vi "Top Level FPGA.vi"() -> ()   [LabVIEW 2012]
uses:
  <vilib>/Platform/TimedLoop/XDataNode/XDataNode.xnode
  <vilib>/Platform/TimedLoop/XDataNode/nitl_modes.ctl
  <vilib>/Platform/TimedLoop/XDataNode/XDNodeRunTimeDep.lvlib
  <vilib>/Platform/TimedLoop/XDataNode/wakeup.ctl
  <vilib>/Platform/TimedLoop/XDataNode/timing_clust.ctl
  <vilib>/rvi/DataTransferAndStorage/Container/Common/niFpgaContainerMetaDataKey.ctl
  <vilib>/rvi/FIFO/Fifo_Types/niFpgaFifoControlLogicControl.ctl
  <vilib>/rvi/Memory/Memory_Types/niFpgaMemoryInterfaceConfiguration.ctl
  <vilib>/rvi/DataTransferAndStorage/Container/Common/niFpgaContainerInitializationParameters.ctl
  <vilib>/rvi/DataTransferAndStorage/Container/Common/niFpgaTransferTypeControl.ctl
  <vilib>/rvi/DataTransferAndStorage/Container/Common/niFpgaContainerArbitrationOptionsControl.ctl
  <vilib>/rvi/DataTransferAndStorage/Container/Common/niFpgaContainerImplementationControl.ctl
  <vilib>/rvi/DataTransferAndStorage/Container/Common/niFpgaDataTypeControl.ctl
  <vilib>/rvi/DataTransferAndStorage/Container/Common/niFpgaContainerState.ctl
  <vilib>/rvi/DataTransferAndStorage/Container/Common/niFpgaContainerSetEmuInfo.vi
  <vilib>/rvi/eio/common/nirviEmuReportErrorAndStop.vi
  <vilib>/rvi/DataTransferAndStorage/Container/Common/niFpgaContainerGetUniqueNameForEmu.vi
  <vilib>/rvi/LocalResourceManager/LocalResourceManager.xnode
  <vilib>/rvi/DataTransferAndStorage/Container/XNode/niFpgaContainer.xnode
  <vilib>/rvi/Memory/Memory_Emulation/nirvimemoryEmulation.vi
  <vilib>/rvi/FIFO/Fifo_Resource/nirvififoEmulationRead.vi
  <vilib>/rvi/FIFO/Fifo_Resource/nirvififoEmulationWrite.vi
  <vilib>/rvi/DataTransferAndStorage/Register/Emulation/niFpgaRegisterEmulation.vi
  <vilib>/eio/EIONode/EIONode.xnode
  <vilib>/rvi/eio/common/nirviEmuTemplateMethod_errors.vi
panel:
  in  "# of pretrigger":u32
  out "IO Module\\Pll Unlocked":bool
  out "IO Module\\ADC Error B":bool
  out "IO Module\\ADC Error A":bool
  out "Init Done":bool
  in  "Simulate":bool
  in  "Trigger 5":i16=12500
  in  "Trigger 6":i16=12500
  in  "Trigger 7":i16=12500
  in  "Trigger 8":i16=12500
  in  "Trigger 3":i16=12500
  in  "Trigger 4":i16=12500
  in  "Trigger 2":i16=12500
  in  "Record Size":u32=300
  in  "Trigger 1":i16=12500
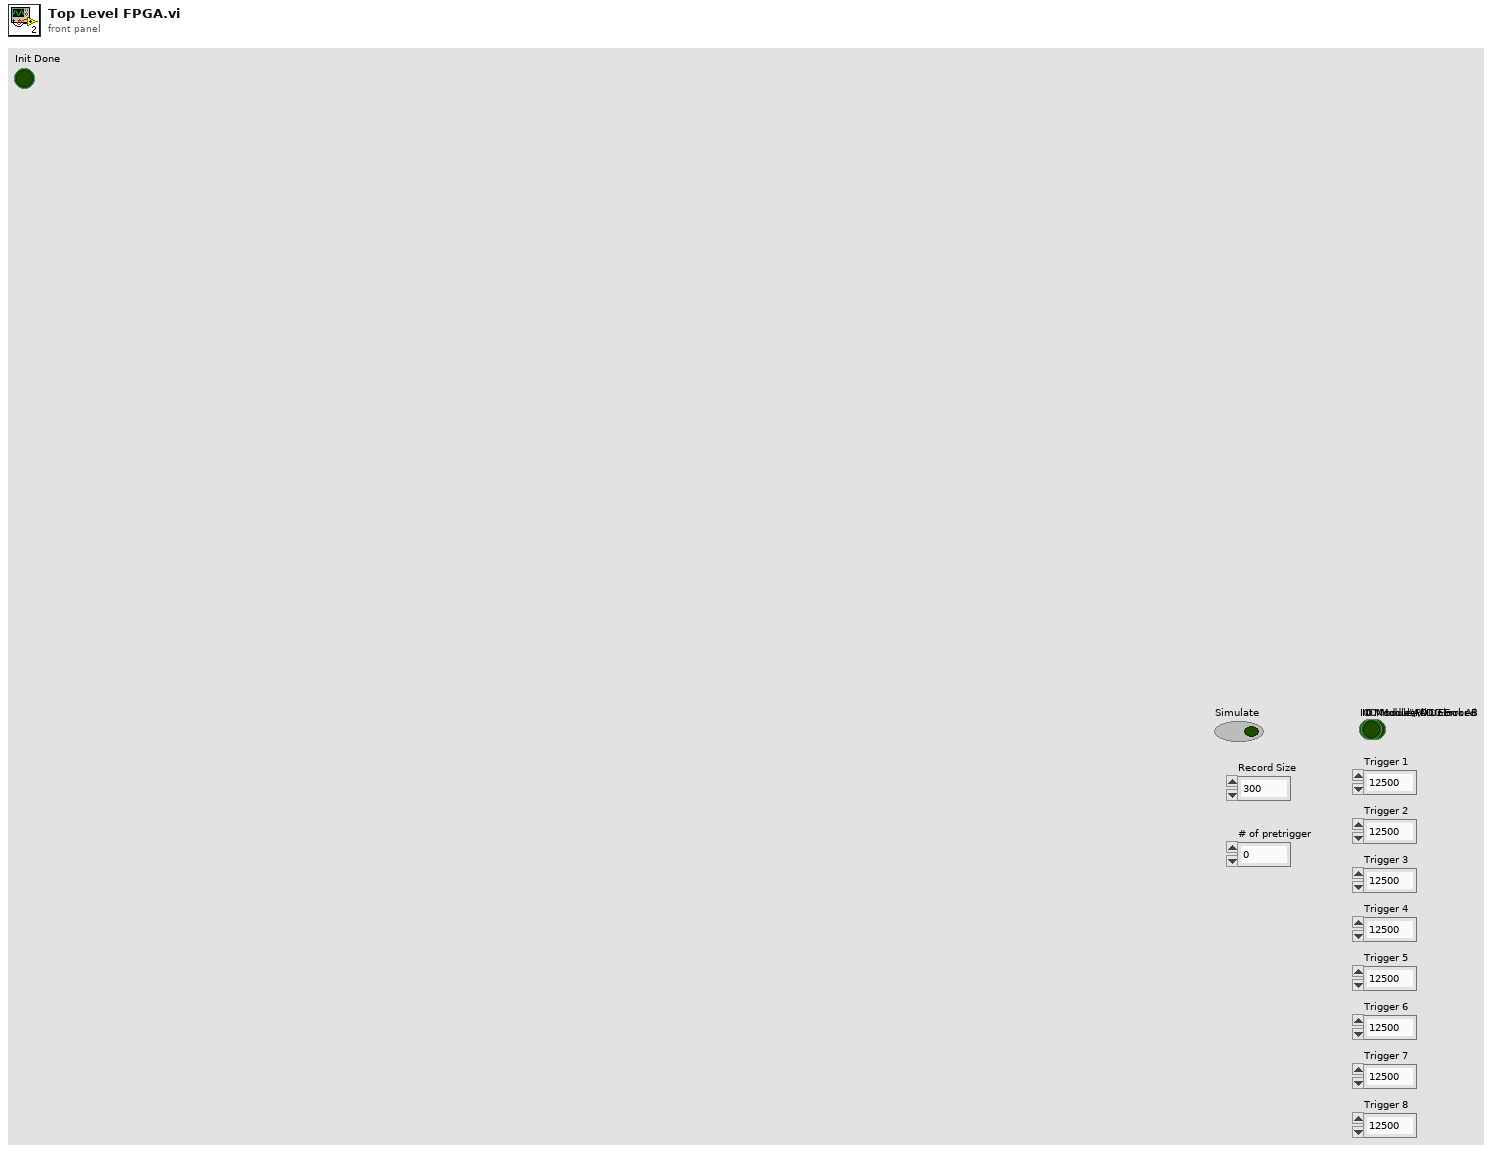
[diagram p1: front panel]
types:
  T1 = typedef "XDNodeRunTimeDep.lvlib/timing_clust.ctl" = cluster{"Expected End [f-1]":u64, "Actual End [f-1]":u64, "Finished Late? [f-1]":bool, "Expected End [i-1]":u64, "Actual End [i-1]":u64, "Finished Late? [i-1]":bool, "Expected Start [i]":u64, "Actual Start [i]":u64, "Expected Start [f]":u64, "Actual Start [f]":u64, "Source Name":string, "Structure Name":string, "Period":i64, "Deadline":i64, "Offset":i64, "Start":i64, "Priority":i32, "Timeout":i32, "Mode":T2, "Wakeup Reason":T3, "Error":errorcluster, "Source Type":string, "Secondary Source Type":string, "Global End Time":u64, "Global Start Time":u64, "Frame Duration":u64, "Iteration Duration":u64, "Assigned CPU":i32, "I/O Scan Engine Mode":u32}
  T2 = typedef "XDNodeRunTimeDep.lvlib/nitl_modes.ctl" = enum32{"No Change", "Process missed periods, maintain original phase", "Discard missed periods, maintain original phase", "Process missed periods, ignore original phase", "Discard missed periods, ignore original phase"}
  T3 = typedef "XDNodeRunTimeDep.lvlib/wakeup.ctl" = enum32{"Normal", "Aborted", "Asynchronous wakeup", "Timing source error", "Timed loop error", "Timeout"}
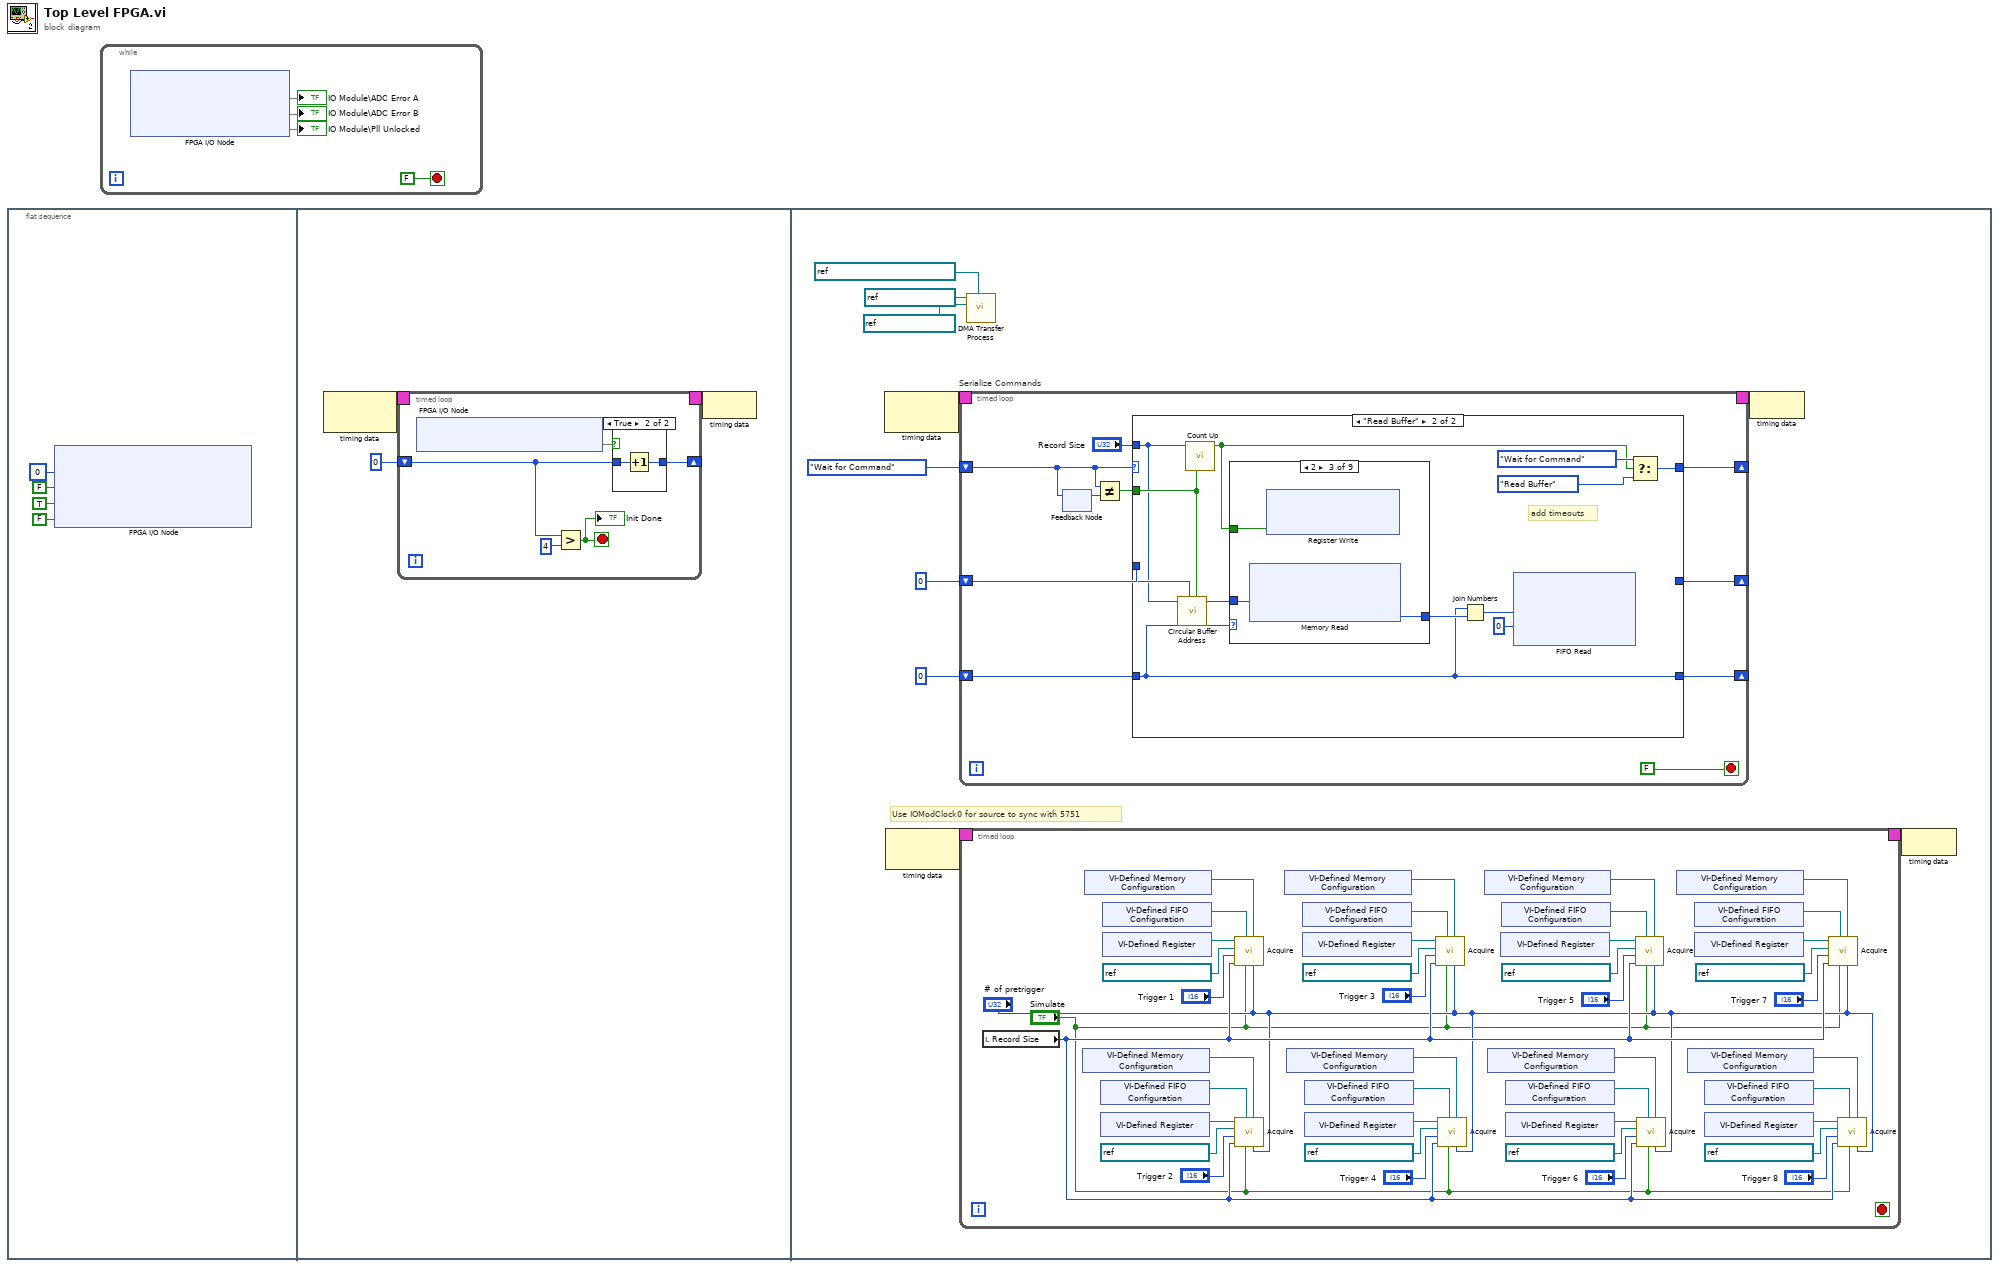
[diagram p0: block diagram]
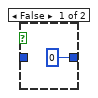
[diagram p2: hidden frame]
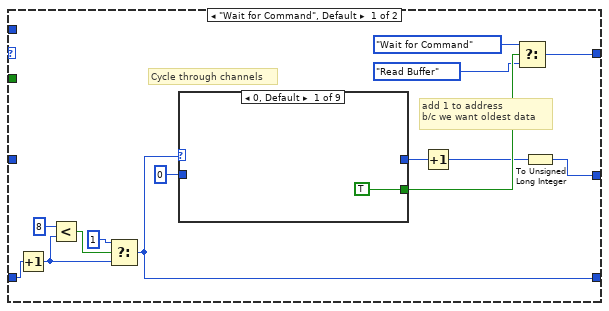
[diagram p3: hidden frame]
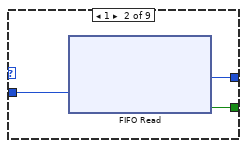
[diagram p4: hidden frame]
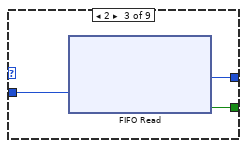
[diagram p5: hidden frame]
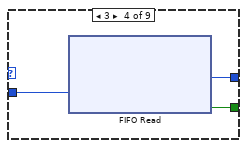
[diagram p6: hidden frame]
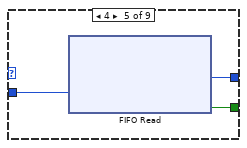
[diagram p7: hidden frame]
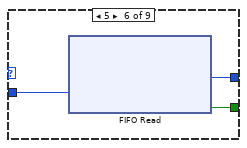
[diagram p8: hidden frame]
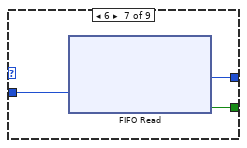
[diagram p9: hidden frame]
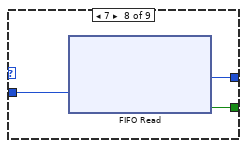
[diagram p10: hidden frame]
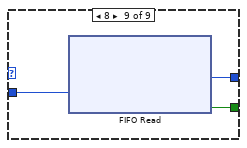
[diagram p11: hidden frame]
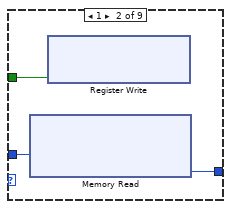
[diagram p13: hidden frame]
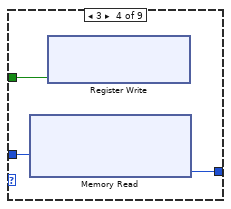
[diagram p14: hidden frame]
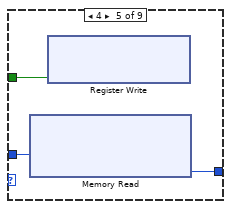
[diagram p15: hidden frame]
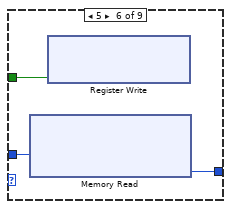
[diagram p16: hidden frame]
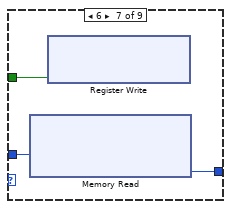
[diagram p17: hidden frame]
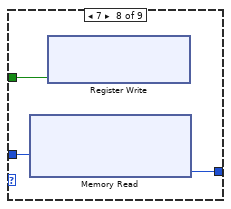
[diagram p18: hidden frame]
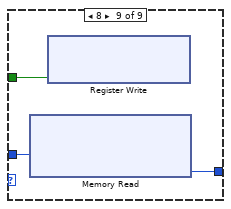
[diagram p19: hidden frame]
diagram:
  n1 = flat-sequence {
    frame #0 {
      n2 = xnode "FPGA I/O Node"("IO Module\\Sample Clock Select"=u8 0 ("IO Module\\Sample Clock Select"), "IO Module\\Force Initialization"=FALSE ("IO Module\\Force Initialization"), "IO Module\\Force Initialization"=TRUE ("IO Module\\Force Initialization"), "IO Module\\Force Initialization"=FALSE ("IO Module\\Force Initialization")) -> ()  [unwired: 4 in, 4 out]
    }
    frame #1 {
      n3 = node-c288() -> (w7:T1)  [unwired: 1 in]
      n4 = timed-loop {
        shift-right: [w11] -> _
        shift-left: u16 0 -> [w10]
        timing: w7 -> [_]
        timing-out: [_] -> w6
        stop <- w8 stop-if-true
        n5 = xnode "FPGA I/O Node"() -> ("IO Module\\Initialization Done"=w12)  [unwired: 1 in, 1 out]
        n6 = Greater?(x=w10, y=u16 4) -> (0:w8:bool)
        "Init Done" <- w8
        n7 = case shown="True" w12 {
          tunnel: [u16 0 w15] -> w11
          tunnel: w10 -> [_ w14]
          frame False {
          }
          frame True {
            n8 = Increment(x=w14) -> (x+1=w15:u16)
          }
        }
      }
      n9 = node-c288(w6) -> ()
    }
    frame #2 {
      # "Use IOModClock0 for source to sync with 5751"
      n10 = node-c288() -> (w27:T1)  [unwired: 1 in]
      n11 = node-c288() -> (w29:T1)  [unwired: 1 in]
      n12 = timed-loop "Serialize Commands" {
        timing: w27 -> [_]
        timing-out: [_] -> w26
        shift-right: [w33] -> _
        shift-left: enum16{"Wait for Command", "Read Buffer"}."Wait for Command" -> [w31]
        shift-right: [w37] -> _
        shift-left: u32 0 ("Element") -> [w36]
        shift-right: [w35] -> _
        shift-left: u8 0 ("t") -> [w34]
        stop <- FALSE stop-if-true
        n13 = feedback-in #1(w31) -> ()
        n14 = feedback #1() -> (w32:enum16{"Wait for Command", "Read Buffer"})  [unwired: 1 in]
        n15 = Not Equal?(x=w31, y=w32) -> (x != y?=w30:bool)
        n16 = case shown="\"Read Buffer\"" w31 {
          tunnel: "Record Size" -> [_ w81]
          tunnel: [w41 w85] -> w35
          tunnel: w34 -> [w43 w85]
          tunnel: [w44 _] -> w37
          tunnel: w36 -> [_ w83]
          tunnel: [w47 w87] -> w33
          tunnel: w30 -> [_ w82]
          frame "Wait for Command", Default {
            # "add 1 to address\nb/c we want oldest data"
            # "Cycle through channels"
            n17 = Increment(x=w43) -> (x+1=w42:u8)
            n18 = Less?(x=u8 8, y=w42) -> (x < y?=w52:bool)
            n19 = Select(t=u8 1, s=w52, f=w42) -> (s? t:f=w41:u8)
            n20 = case shown="0, Default" w41 {
              tunnel: [TRUE ("Timed Out?") w57 w58 w61 w64 w67 w70 w73 w76] -> w48
              tunnel: 0 ("Timeout") -> [_ w56 w60 w63 w66 w69 w72 w75 w78]
              tunnel: [_ w55 w59 w62 w65 w68 w71 w74 w77] -> w49
              frame 0, Default {
              }
              frame 1 {
                n21 = xnode ("FIFO Read")("Timeout"=w56) -> ("Element"=w55:u16, "Timed Out?"=w57:bool)  [unwired: 1 in, 1 out]
              }
              frame 2 {
                n22 = xnode ("FIFO Read")("Timeout"=w60) -> ("Element"=w59:u16, "Timed Out?"=w58:bool)  [unwired: 1 in, 1 out]
              }
              frame 3 {
                n23 = xnode ("FIFO Read")("Timeout"=w63) -> ("Element"=w62:u16, "Timed Out?"=w61:bool)  [unwired: 1 in, 1 out]
              }
              frame 4 {
                n24 = xnode ("FIFO Read")("Timeout"=w66) -> ("Element"=w65:u16, "Timed Out?"=w64:bool)  [unwired: 1 in, 1 out]
              }
              frame 5 {
                n25 = xnode ("FIFO Read")("Timeout"=w69) -> ("Element"=w68:u16, "Timed Out?"=w67:bool)  [unwired: 1 in, 1 out]
              }
              frame 6 {
                n26 = xnode ("FIFO Read")("Timeout"=w72) -> ("Element"=w71:u16, "Timed Out?"=w70:bool)  [unwired: 1 in, 1 out]
              }
              frame 7 {
                n27 = xnode ("FIFO Read")("Timeout"=w75) -> ("Element"=w74:u16, "Timed Out?"=w73:bool)  [unwired: 1 in, 1 out]
              }
              frame 8 {
                n28 = xnode ("FIFO Read")("Timeout"=w78) -> ("Element"=w77:u16, "Timed Out?"=w76:bool)  [unwired: 1 in, 1 out]
              }
            }
            n29 = Increment(x=w49) -> (x+1=w40:u16)
            n30 = Select(t=enum16{"Wait for Command", "Read Buffer"}."Wait for Command", s=w48, f=enum16{"Wait for Command", "Read Buffer"}."Read Buffer") -> (s? t:f=w47:enum16{"Wait for Command", "Read Buffer"})
            n31 = To Unsigned Long Integer(number=w40) -> (unsigned 32bit integer=w44:u32)
          }
          frame "Read Buffer" {
            # "add timeouts"
            n32 = call "Circular Buffer Address.vi"("Reset?"=w82, "Starting Address"=w83, "Records to Acquire"=w81) -> ("Address"=w84:u32)  [unwired: 8 in]
            n33 = call "Count Up.vi"("Reset?"=w82, "goal"=w81) -> ("Count Met"=w79:bool)  [unwired: 8 in, 1 out]
            n34 = case shown="2" w85 {
              tunnel: [_ w92 w95 w98 w101 w104 w107 w110 w113] -> w90
              tunnel: w84 -> [_ w93 w96 w99 w102 w105 w108 w111 w114]
              tunnel: w79 -> [_ w91 w94 w97 w100 w103 w106 w109 w112]
              frame Default {
              }
              frame 1 {
                n35 = xnode ("Memory Read")("Address"=w93) -> ("Data"=w92:i16)  [unwired: 1 in, 1 out]
                n36 = xnode ("Register Write")("Data"=w91) -> ()  [unwired: 1 in, 1 out]
              }
              frame 2 {
                n37 = xnode ("Memory Read")("Address"=w96) -> ("Data"=w95:i16)  [unwired: 1 in, 1 out]
                n38 = xnode ("Register Write")("Data"=w94) -> ()  [unwired: 1 in, 1 out]
              }
              frame 3 {
                n39 = xnode ("Memory Read")("Address"=w99) -> ("Data"=w98:i16)  [unwired: 1 in, 1 out]
                n40 = xnode ("Register Write")("Data"=w97) -> ()  [unwired: 1 in, 1 out]
              }
              frame 4 {
                n41 = xnode ("Memory Read")("Address"=w102) -> ("Data"=w101:i16)  [unwired: 1 in, 1 out]
                n42 = xnode ("Register Write")("Data"=w100) -> ()  [unwired: 1 in, 1 out]
              }
              frame 5 {
                n43 = xnode ("Memory Read")("Address"=w105) -> ("Data"=w104:i16)  [unwired: 1 in, 1 out]
                n44 = xnode ("Register Write")("Data"=w103) -> ()  [unwired: 1 in, 1 out]
              }
              frame 6 {
                n45 = xnode ("Memory Read")("Address"=w108) -> ("Data"=w107:i16)  [unwired: 1 in, 1 out]
                n46 = xnode ("Register Write")("Data"=w106) -> ()  [unwired: 1 in, 1 out]
              }
              frame 7 {
                n47 = xnode ("Memory Read")("Address"=w111) -> ("Data"=w110:i16)  [unwired: 1 in, 1 out]
                n48 = xnode ("Register Write")("Data"=w109) -> ()  [unwired: 1 in, 1 out]
              }
              frame 8 {
                n49 = xnode ("Memory Read")("Address"=w114) -> ("Data"=w113:i16)  [unwired: 1 in, 1 out]
                n50 = xnode ("Register Write")("Data"=w112) -> ()  [unwired: 1 in, 1 out]
              }
            }
            n51 = Join Numbers(hi=w85, lo=w90) -> ((hi.lo)=w86:u32)
            n52 = xnode ("FIFO Read")("Element"=w86, "Timeout"=0) -> ()  [unwired: 1 in, 2 out]
            n53 = Select(t=enum16{"Wait for Command", "Read Buffer"}."Wait for Command", s=w79, f=enum16{"Wait for Command", "Read Buffer"}."Read Buffer") -> (s? t:f=w87:enum16{"Wait for Command", "Read Buffer"})
          }
        }
      }
      n54 = timed-loop {
        timing: w29 -> [_]
        timing-out: [_] -> w28
        stop <- _ stop-if-true
        n55 = local read "Record Size"() -> (w138:u32)
        n56 = xnode "VI-Defined Memory Configuration"() -> ("Memory Out"=w158:refnum<k21>)
        n57 = xnode "VI-Defined Memory Configuration"() -> ("Memory Out"=w119:refnum<k21>)
        n58 = xnode "VI-Defined FIFO Configuration"() -> ("FIFO Out"=w157:refnum<k21>)
        n59 = xnode "VI-Defined Register"() -> ("Register Out"=w135:refnum<k21>)
        n60 = xnode "VI-Defined FIFO Configuration"() -> ("FIFO Out"=w161:refnum<k21>)
        n61 = xnode "VI-Defined Register"() -> ("Register Out"=w137:refnum<k21>)
        n62 = call "Acquire.vi"("# of pretrigger"="# of pretrigger", "Circular Buffer Mem"=w119, "Simulate"="Simulate", "Command FIFO"=w161, "Records to Acquire"=w138, "Trigger"="Trigger 1", "FPGA I/O In"=refnum<k21> "IO Module\\AI A0", "Ch Armed Reg"=w137) -> ()  [unwired: 4 in]
        n63 = call "Acquire.vi"("# of pretrigger"="# of pretrigger", "Circular Buffer Mem"=w158, "Simulate"="Simulate", "Command FIFO"=w157, "Records to Acquire"=w138, "Trigger"="Trigger 2", "FPGA I/O In"=refnum<k21> "IO Module\\AI A1", "Ch Armed Reg"=w135) -> ()  [unwired: 4 in]
        n64 = xnode "VI-Defined Memory Configuration"() -> ("Memory Out"=w152:refnum<k21>)
        n65 = xnode "VI-Defined Memory Configuration"() -> ("Memory Out"=w155:refnum<k21>)
        n66 = xnode "VI-Defined FIFO Configuration"() -> ("FIFO Out"=w151:refnum<k21>)
        n67 = xnode "VI-Defined Register"() -> ("Register Out"=w131:refnum<k21>)
        n68 = xnode "VI-Defined FIFO Configuration"() -> ("FIFO Out"=w156:refnum<k21>)
        n69 = xnode "VI-Defined Register"() -> ("Register Out"=w133:refnum<k21>)
        n70 = call "Acquire.vi"("# of pretrigger"="# of pretrigger", "Circular Buffer Mem"=w152, "Simulate"="Simulate", "Command FIFO"=w151, "Records to Acquire"=w138, "Trigger"="Trigger 3", "FPGA I/O In"=refnum<k21> "IO Module\\AI A2", "Ch Armed Reg"=w131) -> ()  [unwired: 4 in]
        n71 = call "Acquire.vi"("# of pretrigger"="# of pretrigger", "Circular Buffer Mem"=w155, "Simulate"="Simulate", "Command FIFO"=w156, "Records to Acquire"=w138, "Trigger"="Trigger 4", "FPGA I/O In"=refnum<k21> "IO Module\\AI A3", "Ch Armed Reg"=w133) -> ()  [unwired: 4 in]
        n72 = xnode "VI-Defined Memory Configuration"() -> ("Memory Out"=w140:refnum<k21>)
        n73 = xnode "VI-Defined Memory Configuration"() -> ("Memory Out"=w143:refnum<k21>)
        n74 = xnode "VI-Defined Register"() -> ("Register Out"=w125:refnum<k21>)
        n75 = xnode "VI-Defined FIFO Configuration"() -> ("FIFO Out"=w139:refnum<k21>)
        n76 = xnode "VI-Defined FIFO Configuration"() -> ("FIFO Out"=w144:refnum<k21>)
        n77 = xnode "VI-Defined Register"() -> ("Register Out"=w129:refnum<k21>)
        n78 = call "Acquire.vi"("# of pretrigger"="# of pretrigger", "Circular Buffer Mem"=w140, "Simulate"="Simulate", "Command FIFO"=w139, "Records to Acquire"=w138, "Trigger"="Trigger 5", "FPGA I/O In"=refnum<k21> "IO Module\\AI A4", "Ch Armed Reg"=w125) -> ()  [unwired: 4 in]
        n79 = call "Acquire.vi"("# of pretrigger"="# of pretrigger", "Circular Buffer Mem"=w143, "Simulate"="Simulate", "Command FIFO"=w144, "Records to Acquire"=w138, "Trigger"="Trigger 6", "FPGA I/O In"=refnum<k21> "IO Module\\AI A5", "Ch Armed Reg"=w129) -> ()  [unwired: 4 in]
        n80 = xnode "VI-Defined Memory Configuration"() -> ("Memory Out"=w149:refnum<k21>)
        n81 = xnode "VI-Defined Memory Configuration"() -> ("Memory Out"=w146:refnum<k21>)
        n82 = xnode "VI-Defined FIFO Configuration"() -> ("FIFO Out"=w150:refnum<k21>)
        n83 = xnode "VI-Defined Register"() -> ("Register Out"=w127:refnum<k21>)
        n84 = xnode "VI-Defined FIFO Configuration"() -> ("FIFO Out"=w145:refnum<k21>)
        n85 = xnode "VI-Defined Register"() -> ("Register Out"=w123:refnum<k21>)
        n86 = call "Acquire.vi"("# of pretrigger"="# of pretrigger", "Circular Buffer Mem"=w149, "Simulate"="Simulate", "Command FIFO"=w150, "Records to Acquire"=w138, "Trigger"="Trigger 7", "FPGA I/O In"=refnum<k21> "IO Module\\AI A6", "Ch Armed Reg"=w127) -> ()  [unwired: 4 in]
        n87 = call "Acquire.vi"("# of pretrigger"="# of pretrigger", "Circular Buffer Mem"=w146, "Simulate"="Simulate", "Command FIFO"=w145, "Records to Acquire"=w138, "Trigger"="Trigger 8", "FPGA I/O In"=refnum<k21> "IO Module\\AI A7", "Ch Armed Reg"=w123) -> ()  [unwired: 4 in]
      }
      n88 = call "DMA Transfer Process.vi"("Clock Domain"=refnum<k21> "40 MHz Onboard Clock", "Local"=refnum<k21> "To DMA FIFO", "DMA"=refnum<k21> "To Host FIFO") -> ()  [unwired: 9 in]
      n89 = node-c288(w26) -> ()
      n90 = node-c288(w28) -> ()
    }
  }
  n91 = while {
    stop <- FALSE stop-if-true
    n92 = xnode "FPGA I/O Node"() -> ("IO Module\\ADC Error A"=→"IO Module\\ADC Error A", "IO Module\\ADC Error B"=→"IO Module\\ADC Error B", "IO Module\\Pll Unlocked"=→"IO Module\\Pll Unlocked")  [unwired: 3 in, 3 out]
  }
